vi "Point_to_Ponit_distance_measure(subVI).vi"(8 "error in (no error)":errorcluster, 9 "punto finale di misura":i32, 10 "punto di partenza \ndi misura":i32, 11 "Particle Reports (Real-World)":T1(array[cluster]) {"Orientation" format="%.2f"; "Dimensions"."Height" format="%.2f"; "Dimensions"."Width" format="%.2f"; "Center of Mass"."Y" format="%.2f"; "Center of Mass"."X" format="%.2f"; "Bounding Rect"."Bottom" format="%.2f"; "Bounding Rect"."Right" format="%.2f"; "Bounding Rect"."Top" format="%.2f"; "Bounding Rect"."Left" format="%.2f"; "Number of Holes" format="%.2f"; "Area" format="%.2f"}) -> (0 "error out":errorcluster, 3 "distanza tra \ndue i punti (mm)":sgl[](array[numeric]) format="%.4f")   [LabVIEW 2020]
doc: "SUB VI che calcola la distanza tra i centri di massa di du efori identificati da particle reports\n\nin:\nPARTICLE REAPOTS(real word)\nPUNTO DI PARTENZA punto da cui inizio la misura\nPUNTO FINALE punto cui finisce la misura\nERROR IN\n\nout:\nDISTANZA TRA DUE PUNTI(mm)\nERROR OUT"
uses:
  <vilib>/vision/NI_Vision_Development_Module.lvlib
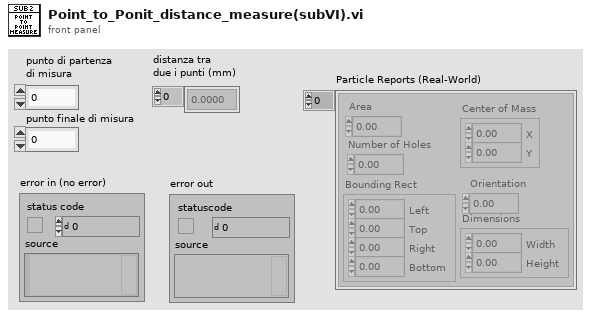
[diagram p1: front panel]
types:
  T1 = cluster{"Area":dbl, "Number of Holes":dbl, "Bounding Rect":cluster{"Left":dbl, "Top":dbl, "Right":dbl, "Bottom":dbl}, "Center of Mass":cluster{"X":dbl, "Y":dbl}, "Orientation":dbl, "Dimensions":cluster{"Width":dbl, "Height":dbl}}[]
  T2 = cluster{"Area":dbl, "Number of Holes":dbl, "Bounding Rect":cluster{"Left":dbl, "Top":dbl, "Right":dbl, "Bottom":dbl}, "Center of Mass":cluster{"X":dbl, "Y":dbl}, "Orientation":dbl, "Dimensions":cluster{"Width":dbl, "Height":dbl}}
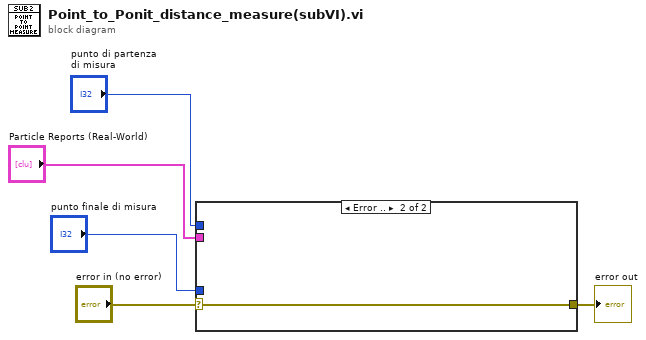
[diagram p0: block diagram]
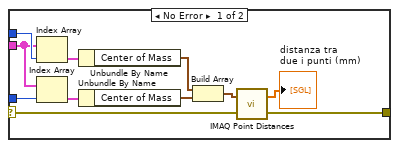
[diagram p2: hidden frame]
diagram:
  n1 = case shown="Error .." "error in (no error)" {
    selector: "error in (no error)" -> [w6 w17]
    tunnel: "punto di partenza \ndi misura" -> [w16 _]
    tunnel: "punto finale di misura" -> [w15 _]
    tunnel: "Particle Reports (Real-World)" -> [w8 _]
    tunnel: [w7 w17] -> w2
    frame No Error {
      n2 = Index Array(array=w8, index=w16) -> (element=w10:T2)
      n3 = Index Array(array=w8, index=w15) -> (element=w9:T2)
      n4 = Unbundle By Name(w10) -> ("Center of Mass"=w13:cluster{"X":dbl, "Y":dbl})
      n5 = Unbundle By Name(w9) -> ("Center of Mass"=w14:cluster{"X":dbl, "Y":dbl})
      n6 = Build Array(w13, w14) -> (w11:cluster{"X":dbl, "Y":dbl}[])
      n7 = call "IMAQ Point Distances"("Points"=w11, "error in (no error)"=w6) -> ("Distances"=→"distanza tra \ndue i punti (mm)":sgl[], "error out"=w7:errorcluster)  [unwired: 3 in]
    }
    frame Error {
    }
  }
  "error out" <- w2
